vi "Initialize Channels.vi"(8 "error in (no error)":errorcluster, 10 "framework configuration":T1, 11 "VeriStand DSF in":refnum<class "VeriStand DSF.lvclass">) -> (0 "error out":errorcluster, 3 "VeriStand DSF out":refnum<class "VeriStand DSF.lvclass">)   [LabVIEW 2017, in "DSF Engine.lvlib" / "VeriStand DSF.lvclass"]
uses:
  VeriStand DSF.lvclass
  DSF Core.lvlibp/Typedefs/DSF Engine Framework Configuration.ctl
  DSF Core.lvlibp/Typedefs/DSF Engine Plugin Configuration.ctl
  DSF Core.lvlibp/Typedefs/DSF Timing Info.ctl
  DSF Core.lvlibp/Typedefs/DSF Engine Plugin Thread Configuration.ctl
  DSF Core.lvlibp/Typedefs/DSF Settings Info.ctl
  DSF Core.lvlibp/Typedefs/DSF Engine Transfer Group Configuration.ctl
  DSF Core.lvlibp/Typedefs/DSF Direction.ctl
  DSF Core.lvlibp/Typedefs/DSF Engine Transfer Configuration.ctl
  DSF Core.lvlibp/Typedefs/DSF Byte Order.ctl
  DSF Core.lvlibp/Typedefs/DSF Engine Channel Configuration.ctl
  DSF Core.lvlibp/Typedefs/DSF Data Type.ctl
  DSF Core.lvlibp/Typedefs/DSF Timeout Behavior.ctl
  DSF Core.lvlibp/Classes/Framework/Framework.lvclass
  <vilib>/NI Veristand/Custom Device API/Custom Device API.lvlib
  C:/Git/DSF/VeriStand/Data Sharing Custom Device/Source/DSF Core.lvlibp/Classes/Framework/Framework.lvclass
  DSF Core.lvlibp
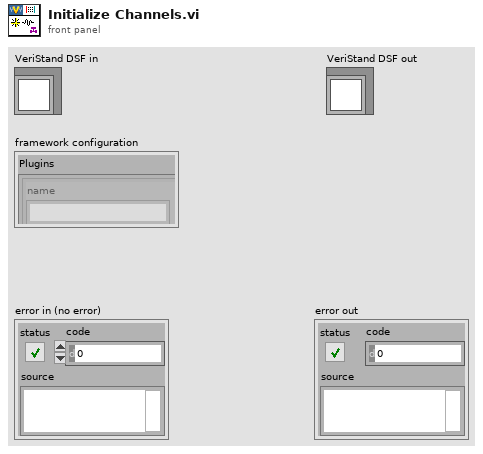
[diagram p1: front panel]
types:
  T1 = typedef "DSF Core.lvlibp/DSF Engine Framework Configuration.ctl" = cluster{"Plugins":T2[]}
  T2 = typedef "DSF Core.lvlibp/DSF Engine Plugin Configuration.ctl" = cluster{"name":string, "components":string[], "cycle timing":T3, "threads":T4[], "Transfer Groups":T6[], "settings":T5}
  T3 = typedef "DSF Core.lvlibp/DSF Timing Info.ctl" = cluster{"priority":u64, "decimation":u64, "offset":u64}
  T4 = typedef "DSF Core.lvlibp/DSF Engine Plugin Thread Configuration.ctl" = cluster{"buffer converter settings":T5, "transceiver settings":T5, "custom settings":T5, "processor":i32, "priority offset":i16}
  T5 = typedef "DSF Core.lvlibp/DSF Settings Info.ctl" = cluster{"key":string, "value":string}[]
  T6 = typedef "DSF Core.lvlibp/DSF Engine Transfer Group Configuration.ctl" = cluster{"name":string, "direction":T7, "cycle timing":T3, "thread index":i32, "settings":T5, "Transfers":T8[], "timeout behavior":T12}
  T7 = typedef "DSF Core.lvlibp/DSF Direction.ctl" = enum8{"Tx", "Rx"}
  T8 = typedef "DSF Core.lvlibp/DSF Engine Transfer Configuration.ctl" = cluster{"name":string, "byte order":T9, "settings":T5, "channels":T10[]}
  T9 = typedef "DSF Core.lvlibp/DSF Byte Order.ctl" = enum8{"big-endian", "little-endian"}
  T10 = typedef "DSF Core.lvlibp/DSF Engine Channel Configuration.ctl" = cluster{"string offset":u64, "string data type":T11, "engine data type":T11, "name":string, "settings":T5, "units":string}
  T11 = typedef "DSF Core.lvlibp/DSF Data Type.ctl" = enum8{"Bool", "SGL", "DBL", "I8", "I16", "I32", "I64", "U8", "U16", "U32", "U64"}
  T12 = typedef "DSF Core.lvlibp/DSF Timeout Behavior.ctl" = enum8{"Increment Late Count", "Throw Error"}
  T13 = enum16{"open", "replace", "create", "open or create", "replace or create", "replace or create with confirmation"}
  T14 = typedef "Custom Device API.lvlib/Custom Device Item Ref.ctl" = u64
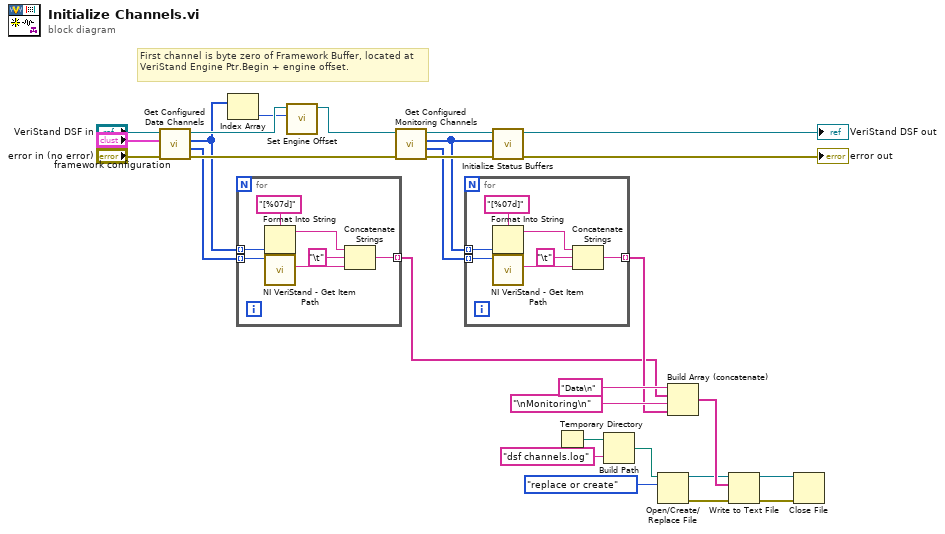
[diagram p0: block diagram]
diagram:
  # "First channel is byte zero of Framework Buffer, located at VeriStand Engine Ptr.Begin + engine offset."
  n1 = call "Get Configured Data Channels.vi"("error in (no error)"="error in (no error)", "framework configuration"="framework configuration", "VeriStand Data Sharing Framework in"="VeriStand DSF in") -> ("error out"=w14:errorcluster, "data channels refs"=w2:T14[], "data channel offsets"=w3:u64[], "VeriStand Data Sharing Framework out"=w11:refnum<class "VeriStand DSF.lvclass">)  [unwired: 5 in]
  n2 = Index Array(array=w3) -> (element=w10:u64)  [unwired: 1 in]
  n3 = for {
    tunnel: [w33] -> w1 mode=indexing
    tunnel: w3 -> [w29] mode=indexing
    tunnel: w2 -> [w32] mode=indexing
    n4 = Format Into String(format string="[%07d]", w29) -> (resulting string=w30:string)  [unwired: 2 in, 1 out]
    n5 = call <vilib>:"NI VeriStand - Get Item Path.vi"("Item Ref in"=w32) -> ("Path"=w34:string)  [unwired: 7 in, 3 out]
    n6 = Concatenate Strings(w30, "\t" ("string"), w34) -> (w33:string)
  }
  n7 = call "Set Engine Offset.vi"("engine offset"=w10, "Framework in"=w11) -> ("Framework out"=w15:refnum<class "VeriStand DSF.lvclass">)  [unwired: 9 in]
  n8 = call "Get Configured Monitoring Channels.vi"("error in (no error)"=w14, "VeriStand Data Sharing Framework in"=w15) -> ("error out"=w17:errorcluster, "monitoring channels refs"=w4:T14[], "monitoring channel offsets"=w6:u64[], "VeriStand Data Sharing Framework out"=w16:refnum<class "VeriStand DSF.lvclass">)  [unwired: 6 in]
  n9 = for {
    tunnel: [w39] -> w8 mode=indexing
    tunnel: w6 -> [w36] mode=indexing
    tunnel: w4 -> [w41] mode=indexing
    n10 = Format Into String(format string="[%07d]", w36) -> (resulting string=w37:string)  [unwired: 2 in, 1 out]
    n11 = call <vilib>:"NI VeriStand - Get Item Path.vi"("Item Ref in"=w41) -> ("Path"=w40:string)  [unwired: 7 in, 3 out]
    n12 = Concatenate Strings(w37, "\t" ("string"), w40) -> (w39:string)
  }
  n13 = call "Initialize Status Buffers.vi"("error in (no error)"=w17, "monitoring channel offsets"=w6, "VeriStand DSF in"=w16) -> ("error out"=→"error out":errorcluster, "VeriStand DSF out"=→"VeriStand DSF out":refnum<class "VeriStand DSF.lvclass">)  [unwired: 7 in]
  n14 = Temporary Directory() -> (w19:path)
  n15 = Build Path(base path=w19, name or relative path="dsf channels.log") -> (appended path=w21:path)
  n16 = Open/Create/Replace File(file path (use dialog)=w21, operation (0:open)=T13."replace or create") -> (refnum out=w22:refnum<file>, error out=w23:errorcluster)  [unwired: 4 in, 1 out]
  n17 = Build Array (concatenate)("Data\n", w1, "\nMonitoring\n", w8) -> (w28:string[])
  n18 = Write to Text File(file (use dialog)=w22, text=w28, error in=w23) -> (refnum out=w25:refnum<file>, error out=w24:errorcluster)  [unwired: 1 in, 1 out]
  n19 = Close File(refnum=w25, error in=w24) -> ()  [unwired: 2 out]
